vi "Three_Tote_Before_Encoder_Added.vi"(11 "3_Tote_Enable":bool=TRUE) -> ()   [LabVIEW 2014]
uses:
  General_VI/Global Var.vi
panel:
  in  "Time _To_Drive_1_Tote":i32=8000
  in  "Extend_Flipper_Time":i32=500
  in  "Open_Infeed_time":i32=800
  # "Static Tunning Values"
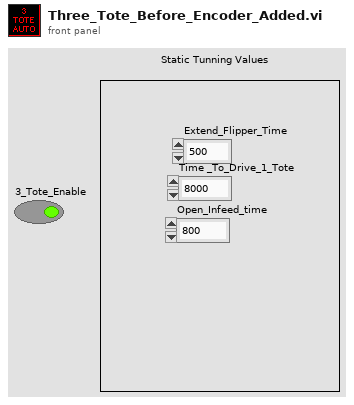
[diagram p1: front panel]
types:
  T1 = cluster{"Open_Infeed_time":i32, "Extend_Flipper_Time":i32, "Time _To_Drive_1_Tote":i32}
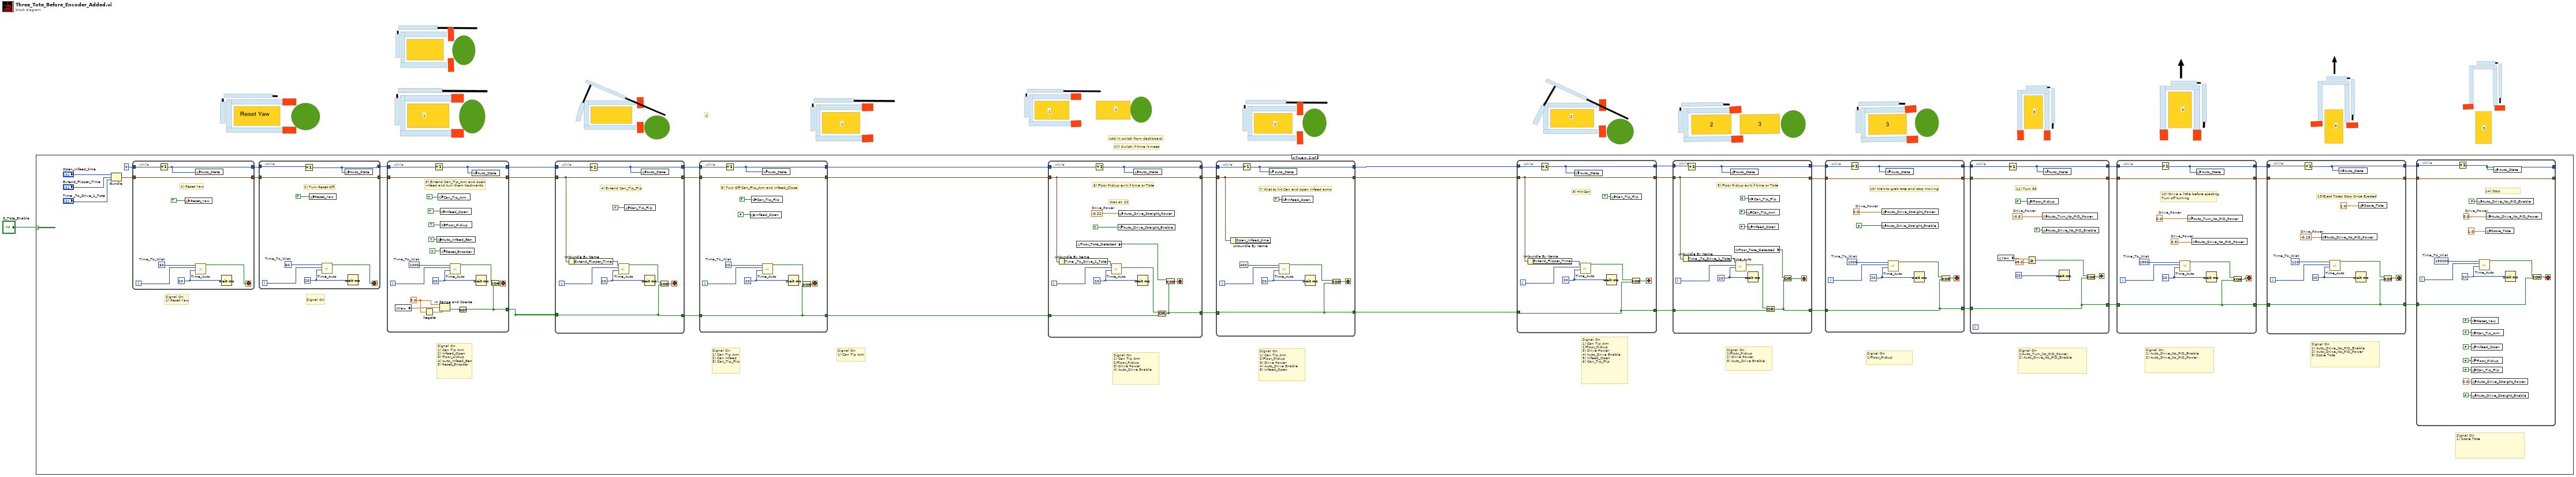
[diagram p0: block diagram]
diagram:
  # "3"
  # "3"
  # "3"
  # "3"
  # "2"
  # "2"
  # "2"
  # "1"
  # "1"
  # "1"
  # "1"
  # "Add in switch from dashboard"
  # "Kill Switch if time it meet"
  n1 = case shown="True" "3_Tote_Enable" {
    frame False {
    }
    frame True {
      # "Signal On\n1) Score Tote"
      # "Signal On\n1) Auto_Drive_No_PID_Enable\n2) Auto_Drive_No_PID_Power\n3) Score Tote"
      # "Signal On\n1) Auto_Drive_No_PID_Enable\n2) Auto_Drive_No_PID_Power"
      # "Signal On\n1)Auto_Turn_No_PID_Power\n2) Auto_Drive_No_PID_Enable"
      # "Signal On\n1)Floor_Pickup"
      # "Signal On\n1)Floor_Pickup\n2) Drive Power\n3) Auto_Drive Enable"
      # "Signal On\n1) Can Tip Arm\n2)Floor_Pickup\n3) Drive Power\n4) Auto_Drive Enable\n5) Infeed_Open\n6) Can_Tip_Flip"
      # "Signal On\n1) Can Tip Arm\n2)Floor_Pickup\n3) Drive Power\n4) Auto_Drive Enable\n5) Infeed_Open"
      # "Signal On\n1) Can Tip Arm\n2)Floor_Pickup\n3) Drive Power\n4) Auto_Drive Enable"
      # "Signal On\n1) Can Tip Arm"
      # "Signal On\n1) Can Tip Arm\n2) Can Infeed\n3) Can_Tip_Flip"
      # "Signal On\n1) Can Tip Arm\n2) Infeed_Open\n3) Floor_pickup\n4) Auto_Infeed_Ben\n5) Reset_Encoder"
      # "Signal On"
      # "Signal On\n1) Reset Yaw"
      n2 = Bundle("Open_Infeed_time"="Open_Infeed_time", "Extend_Flipper_Time"="Extend_Flipper_Time", "Time _To_Drive_1_Tote"="Time _To_Drive_1_Tote") -> (w27:T1)  [unwired: 1 in]
      n3 = while {
        tunnel: 0 -> [w203]
        tunnel: [w202] -> w42
        tunnel: w27 -> [w204]
        tunnel: [w204] -> w26
        i -> [w207]
        stop <- w209 stop-if-true
        w208 = u32 20 ("milliseconds to wait")
        w206 = 60  # Time_To_Wiat
        # "1) Reset Yaw"
        n4 = Increment(x=w203) -> (x+1=w202:i32)
        n5 = global write "Global Var.vi" "Reset_Yaw"(TRUE) -> ()
        n6 = global write "Global Var.vi" "Auto_State"(w202) -> ()
        n7 = call "Time_Auto.vi"("Sample_Time"=w208, "Counter"=w207, "Time_to_wait"=w206) -> ("Boolean"=w209:bool)  [unwired: 8 in]
        n8 = Wait (ms)(milliseconds to wait=w208) -> ()  [unwired: 1 out]
      }
      n9 = while {
        tunnel: w42 -> [w195]
        tunnel: [w194] -> w41
        tunnel: w26 -> [w196]
        tunnel: [w196] -> w25
        i -> [w199]
        stop <- w201 stop-if-true
        w200 = u32 20 ("milliseconds to wait")
        w198 = 60  # Time_To_Wiat
        # "2) Turn Reset Off"
        n10 = Increment(x=w195) -> (x+1=w194:i32)
        n11 = global write "Global Var.vi" "Reset_Yaw"(FALSE) -> ()
        n12 = call "Time_Auto.vi"("Sample_Time"=w200, "Counter"=w199, "Time_to_wait"=w198) -> ("Boolean"=w201:bool)  [unwired: 8 in]
        n13 = global write "Global Var.vi" "Auto_State"(w194) -> ()
        n14 = Wait (ms)(milliseconds to wait=w200) -> ()  [unwired: 1 out]
      }
      n15 = while {
        tunnel: w41 -> [w188]
        tunnel: [w187] -> w14
        tunnel: w25 -> [w189]
        tunnel: [w189] -> w13
        tunnel: [w178] -> w12
        i -> [w192]
        stop <- w180 stop-if-true
        w182 = 5.0 ("upper limit")
        w193 = u32 20 ("milliseconds to wait")
        w191 = 1000  # Time_To_Wiat
        # "3) Extend Can_Tip_Arm and open \ninfeed and turn them backwards"
        n16 = global read "Global Var.vi" "Yaw"() -> (w184:dbl)
        n17 = Negate(x=w182) -> (-x=w183:dbl)
        n18 = Increment(x=w188) -> (x+1=w187:i32)
        n19 = global write "Global Var.vi" "Auto_Infeed_Ben"(TRUE) -> ()
        n20 = global write "Global Var.vi" "Can_Tip_Arm"(TRUE) -> ()
        n21 = In Range and Coerce(upper limit=w182, x=w184, lower limit=w183) -> (In Range?=w179:bool)  [unwired: 1 out]
        n22 = global write "Global Var.vi" "Infeed_Open"(TRUE) -> ()
        n23 = global write "Global Var.vi" "Floor_Pickup"(TRUE) -> ()
        n24 = global write "Global Var.vi" "Reset_Encoder"(TRUE) -> ()
        n25 = call "Time_Auto.vi"("Sample_Time"=w193, "Counter"=w192, "Time_to_wait"=w191) -> ("Boolean"=w181:bool)  [unwired: 8 in]
        n26 = Not(x=w179) -> (.not. x?=w178:bool)
        n27 = global write "Global Var.vi" "Auto_State"(w187) -> ()
        n28 = Wait (ms)(milliseconds to wait=w193) -> ()  [unwired: 1 out]
        n29 = Exclusive Or(1:w178, 2:w181) -> (0:w180:bool)
      }
      n30 = while {
        tunnel: w14 -> [w172]
        tunnel: [w171] -> w40
        tunnel: w13 -> [w170]
        tunnel: [w170] -> w24
        tunnel: w12 -> [_]
        tunnel: w12 -> [w166]
        tunnel: [w166] -> w11
        i -> [w174]
        stop <- w168 stop-if-true
        w175 = u32 20 ("milliseconds to wait")
        # "4) Extend Can_Tip_Flip"
        n31 = Unbundle By Name(w170) -> ("Extend_Flipper_Time"=w169:i32)
        n32 = Increment(x=w172) -> (x+1=w171:i32)
        n33 = call "Time_Auto.vi"("Sample_Time"=w175, "Counter"=w174, "Time_to_wait"=w169) -> ("Boolean"=w167:bool)  [unwired: 8 in]
        n34 = global write "Global Var.vi" "Can_Tip_Flip"(TRUE) -> ()
        n35 = global write "Global Var.vi" "Auto_State"(w171) -> ()
        n36 = Wait (ms)(milliseconds to wait=w175) -> ()  [unwired: 1 out]
        n37 = Exclusive Or(1:w166, 2:w167) -> (0:w168:bool)
      }
      n38 = while {
        tunnel: w40 -> [w159]
        tunnel: [w158] -> w36
        tunnel: w24 -> [w160]
        tunnel: [w160] -> w23
        tunnel: w11 -> [w155]
        tunnel: [w155] -> w10
        i -> [w164]
        stop <- w157 stop-if-true
        w165 = u32 20 ("milliseconds to wait")
        w163 = 20  # Time_To_Wiat
        # "5) Turn Off Can_Flip_Arm and Infeed_Close"
        n39 = Increment(x=w159) -> (x+1=w158:i32)
        n40 = global write "Global Var.vi" "Infeed_Open"(FALSE) -> ()
        n41 = global write "Global Var.vi" "Can_Tip_Flip"(FALSE) -> ()
        n42 = call "Time_Auto.vi"("Sample_Time"=w165, "Counter"=w164, "Time_to_wait"=w163) -> ("Boolean"=w156:bool)  [unwired: 8 in]
        n43 = global write "Global Var.vi" "Auto_State"(w158) -> ()
        n44 = Wait (ms)(milliseconds to wait=w165) -> ()  [unwired: 1 out]
        n45 = Exclusive Or(1:w155, 2:w156) -> (0:w157:bool)
      }
      n46 = while {
        tunnel: w36 -> [w152]
        tunnel: [w151] -> w39
        tunnel: w23 -> [w150]
        tunnel: [w150] -> w22
        tunnel: w10 -> [w146]
        tunnel: [w142] -> w9
        i -> [w153]
        stop <- w143 stop-if-true
        w148 = -0.22  # Drive_Power
        w154 = u32 20 ("milliseconds to wait")
        # "Was at .22"
        # "6) Floor Pickup exit if time or Tote"
        n47 = Unbundle By Name(w150) -> ("Time _To_Drive_1_Tote"=w149:i32)
        n48 = global read "Global Var.vi" "Floor_Tote_Detected"() -> (w144:bool)
        n49 = Increment(x=w152) -> (x+1=w151:i32)
        n50 = call "Time_Auto.vi"("Sample_Time"=w154, "Counter"=w153, "Time_to_wait"=w149) -> ("Boolean"=w145:bool)  [unwired: 8 in]
        n51 = global write "Global Var.vi" "Auto_Drive_Straight_Enable"(TRUE) -> ()
        n52 = global write "Global Var.vi" "Auto_Drive_Straight_Power"(w148) -> ()
        n53 = global write "Global Var.vi" "Auto_State"(w151) -> ()
        n54 = Wait (ms)(milliseconds to wait=w154) -> ()  [unwired: 1 out]
        n55 = Compound Arithmetic op=OR(w145, w146) -> (w142:bool)
        n56 = Exclusive Or(1:w142, 2:w144) -> (0:w143:bool)
      }
      n57 = while {
        tunnel: w39 -> [w138]
        tunnel: [w137] -> w35
        tunnel: w22 -> [w136]
        tunnel: [w136] -> w21
        tunnel: w9 -> [w132]
        tunnel: [w132] -> w8
        i -> [w140]
        stop <- w134 stop-if-true
        w141 = u32 20 ("milliseconds to wait")
        # "7) Wiat to hit Can and open infeed arms"
        n58 = Unbundle By Name(w136) -> ()  [unwired: 1 out]
        n59 = Increment(x=w138) -> (x+1=w137:i32)
        n60 = global write "Global Var.vi" "Auto_State"(w137) -> ()
        n61 = call "Time_Auto.vi"("Sample_Time"=w141, "Counter"=w140, "Time_to_wait"=400) -> ("Boolean"=w133:bool)  [unwired: 8 in]
        n62 = global write "Global Var.vi" "Infeed_Open"(TRUE ("Infeed_Open")) -> ()
        n63 = Wait (ms)(milliseconds to wait=w141) -> ()  [unwired: 1 out]
        n64 = Exclusive Or(1:w132, 2:w133) -> (0:w134:bool)
      }
      n65 = while {
        tunnel: w35 -> [w128]
        tunnel: [w127] -> w38
        tunnel: w21 -> [w126]
        tunnel: [w126] -> w20
        tunnel: w8 -> [w122]
        tunnel: [w122] -> w7
        i -> [w130]
        stop <- w123 stop-if-true
        w131 = u32 20 ("milliseconds to wait")
        # "8) HIt Can"
        n66 = Unbundle By Name(w126) -> ("Extend_Flipper_Time"=w125:i32)
        n67 = Increment(x=w128) -> (x+1=w127:i32)
        n68 = global write "Global Var.vi" "Auto_State"(w127) -> ()
        n69 = call "Time_Auto.vi"("Sample_Time"=w131, "Counter"=w130, "Time_to_wait"=w125) -> ("Boolean"=w124:bool)  [unwired: 8 in]
        n70 = Wait (ms)(milliseconds to wait=w131) -> ()  [unwired: 1 out]
        n71 = global write "Global Var.vi" "Can_Tip_Flip"(TRUE ("Infeed_Open")) -> ()
        n72 = Exclusive Or(1:w122, 2:w124) -> (0:w123:bool)
      }
      n73 = while {
        tunnel: w38 -> [w114]
        tunnel: [w113] -> w37
        tunnel: w20 -> [w111]
        tunnel: [w111] -> w19
        tunnel: w7 -> [w110]
        tunnel: [w108] -> w6
        i -> [w120]
        stop <- w119 stop-if-true
        w121 = u32 20 ("milliseconds to wait")
        # "9) Floor Pickup exit if time or Tote"
        n74 = Unbundle By Name(w111) -> ("Time _To_Drive_1_Tote"=w112:i32)
        n75 = Increment(x=w114) -> (x+1=w113:i32)
        n76 = global write "Global Var.vi" "Auto_State"(w113) -> ()
        n77 = global read "Global Var.vi" "Floor_Tote_Detected"() -> (w118:bool)
        n78 = call "Time_Auto.vi"("Sample_Time"=w121, "Counter"=w120, "Time_to_wait"=w112) -> ("Boolean"=w109:bool)  [unwired: 8 in]
        n79 = global write "Global Var.vi" "Can_Tip_Arm"(FALSE ("Infeed_Open")) -> ()
        n80 = global write "Global Var.vi" "Infeed_Open"(FALSE ("Infeed_Open")) -> ()
        n81 = Wait (ms)(milliseconds to wait=w121) -> ()  [unwired: 1 out]
        n82 = global write "Global Var.vi" "Can_Tip_Flip"(FALSE ("Infeed_Open")) -> ()
        n83 = Compound Arithmetic op=OR(w109, w110) -> (w108:bool)
        n84 = Or(x=w118, y=w108) -> (x .or. y?=w119:bool)
      }
      n85 = while {
        tunnel: w37 -> [w103]
        tunnel: [w102] -> w34
        tunnel: w19 -> [w104]
        tunnel: [w104] -> w18
        tunnel: w6 -> [w97]
        tunnel: [w97] -> w5
        i -> [w106]
        stop <- w99 stop-if-true
        w101 = 0.0  # Drive_Power
        w107 = u32 20 ("milliseconds to wait")
        w105 = 1000  # Time_To_Wiat
        # "10) Wait to grab tote and stop moving"
        n86 = Increment(x=w103) -> (x+1=w102:i32)
        n87 = global write "Global Var.vi" "Auto_Drive_Straight_Enable"(FALSE) -> ()
        n88 = global write "Global Var.vi" "Auto_Drive_Straight_Power"(w101) -> ()
        n89 = global write "Global Var.vi" "Auto_State"(w102) -> ()
        n90 = call "Time_Auto.vi"("Sample_Time"=w107, "Counter"=w106, "Time_to_wait"=w105) -> ("Boolean"=w98:bool)  [unwired: 8 in]
        n91 = Wait (ms)(milliseconds to wait=w107) -> ()  [unwired: 1 out]
        n92 = Exclusive Or(1:w97, 2:w98) -> (0:w99:bool)
      }
      n93 = while {
        tunnel: w34 -> [w91]
        tunnel: [w90] -> w33
        tunnel: w18 -> [w92]
        tunnel: [w92] -> w17
        tunnel: w5 -> [w85]
        tunnel: [w85] -> w4
        stop <- w87 stop-if-true
        w89 = -0.6  # Drive_Power
        # "11) Turn 90"
        n94 = global read "Global Var.vi" "Yaw"() -> (w94:dbl)
        n95 = Increment(x=w91) -> (x+1=w90:i32)
        n96 = Greater Or Equal?(x=w94, y=48.0) -> (x >= y?=w86:bool)
        n97 = global write "Global Var.vi" "Floor_Pickup"(FALSE) -> ()
        n98 = global write "Global Var.vi" "Auto_Turn_No_PID_Power"(w89) -> ()
        n99 = global write "Global Var.vi" "Auto_Drive_No_PID_Enable"(TRUE ("Auto_Drive_No_PID_Enable")) -> ()
        n100 = global write "Global Var.vi" "Auto_State"(w90) -> ()
        n101 = Wait (ms)(milliseconds to wait=u32 20) -> ()  [unwired: 1 out]
        n102 = Exclusive Or(1:w85, 2:w86) -> (0:w87:bool)
      }
      n103 = while {
        tunnel: w33 -> [w79]
        tunnel: [w78] -> w32
        tunnel: w17 -> [w80]
        tunnel: [w80] -> w16
        tunnel: w4 -> [w74]
        tunnel: [w74] -> w3
        i -> [w83]
        stop <- w76 stop-if-true
        w77 = 0.0  # Drive_Power
        w81 = 0.5  # Drive_Power
        w84 = u32 20 ("milliseconds to wait")
        w82 = 1900  # Time_To_Wiat
        # "12) Drive a little before ejecting\nTurn off turning"
        n104 = Increment(x=w79) -> (x+1=w78:i32)
        n105 = call "Time_Auto.vi"("Sample_Time"=w84, "Counter"=w83, "Time_to_wait"=w82) -> ("Boolean"=w75:bool)  [unwired: 8 in]
        n106 = global write "Global Var.vi" "Auto_Turn_No_PID_Power"(w77) -> ()
        n107 = global write "Global Var.vi" "Auto_Drive_No_PID_Power"(w81) -> ()
        n108 = global write "Global Var.vi" "Auto_State"(w78) -> ()
        n109 = Wait (ms)(milliseconds to wait=w84) -> ()  [unwired: 1 out]
        n110 = Exclusive Or(1:w74, 2:w75) -> (0:w76:bool)
      }
      n111 = while {
        tunnel: w32 -> [w68]
        tunnel: [w67] -> w31
        tunnel: w16 -> [w69]
        tunnel: [w69] -> w15
        tunnel: w3 -> [w63]
        tunnel: [w63] -> w2
        i -> [w72]
        stop <- w65 stop-if-true
        w66 = -0.15  # Drive_Power
        w73 = u32 20 ("milliseconds to wait")
        w71 = 120  # Time_To_Wiat
        # "13)Eject Totes Stop Once Ejected"
        n112 = Increment(x=w68) -> (x+1=w67:i32)
        n113 = global write "Global Var.vi" "Auto_Drive_No_PID_Power"(w66) -> ()
        n114 = call "Time_Auto.vi"("Sample_Time"=w73, "Counter"=w72, "Time_to_wait"=w71) -> ("Boolean"=w64:bool)  [unwired: 8 in]
        n115 = global write "Global Var.vi" "Auto_State"(w67) -> ()
        n116 = Wait (ms)(milliseconds to wait=w73) -> ()  [unwired: 1 out]
        n117 = global write "Global Var.vi" "Score_Tote"(1.0) -> ()
        n118 = Exclusive Or(1:w63, 2:w64) -> (0:w65:bool)
      }
      n119 = while {
        tunnel: w31 -> [w57]
        tunnel: w15 -> [w58]
        tunnel: [w58] -> _
        tunnel: [w56] -> _
        tunnel: w2 -> [w51]
        i -> [w61]
        stop <- w53 stop-if-true
        w54 = 0.0  # Drive_Power
        w62 = u32 20 ("milliseconds to wait")
        w60 = 150000  # Time_To_Wiat
        # "14) Stop"
        n120 = Increment(x=w57) -> (x+1=w56:i32)
        n121 = global write "Global Var.vi" "Reset_Yaw"(FALSE ("Reset_Yaw")) -> ()
        n122 = global write "Global Var.vi" "Can_Tip_Arm"(FALSE ("Can_Tip_Arm")) -> ()
        n123 = global write "Global Var.vi" "Infeed_Open"(FALSE ("Infeed_Open")) -> ()
        n124 = global write "Global Var.vi" "Floor_Pickup"(FALSE ("Floor_Pickup")) -> ()
        n125 = global write "Global Var.vi" "Can_Tip_Flip"(FALSE ("Can_Tip_Flip")) -> ()
        n126 = global write "Global Var.vi" "Auto_Drive_Straight_Enable"(FALSE ("Auto_Drive_Straight_Enable")) -> ()
        n127 = global write "Global Var.vi" "Auto_Drive_Straight_Power"(0.0 ("Auto_Drive_Straight_Power")) -> ()
        n128 = global write "Global Var.vi" "Auto_Drive_No_PID_Enable"(FALSE ("Auto_Drive_No_PID_Enable")) -> ()
        n129 = call "Time_Auto.vi"("Sample_Time"=w62, "Counter"=w61, "Time_to_wait"=w60) -> ("Boolean"=w52:bool)  [unwired: 8 in]
        n130 = global write "Global Var.vi" "Score_Tote"(1.0) -> ()
        n131 = global write "Global Var.vi" "Auto_Drive_No_PID_Power"(w54) -> ()
        n132 = global write "Global Var.vi" "Auto_State"(w56) -> ()
        n133 = Wait (ms)(milliseconds to wait=w62) -> ()  [unwired: 1 out]
        n134 = Exclusive Or(1:w51, 2:w52) -> (0:w53:bool)
      }
    }
  }
